vi "index-i8.vi"(9 "长度":i32, 10 "索引":i32, 11 "数组":u8[](array[numeric])) -> (3 "数值输出":i8)   [LabVIEW 2012]
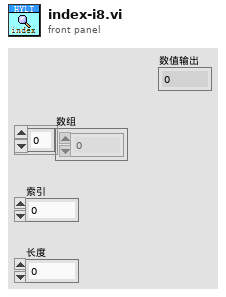
[diagram p1: front panel]
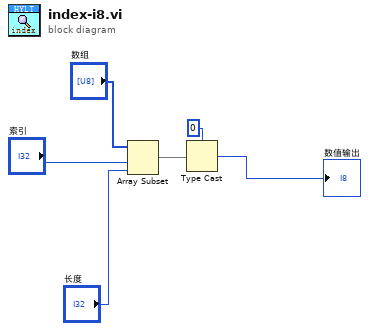
[diagram p0: block diagram]
diagram:
  n1 = Array Subset(array="数组", index="索引", length="长度") -> (w3:u8[])
  n2 = Type Cast(type=i8 0 ("数值输入"), x=w3) -> (*(type *) &x=→"数值输出":i8)
